vi "生成二维坐标点.vi"(1 "输入无序一维坐标点":cluster{"X":sgl, "Y":sgl}[](array[cluster])) -> (0 "输出有序二维坐标点":cluster{"X":sgl, "Y":sgl}[][](array[cluster]))   [LabVIEW 2018]
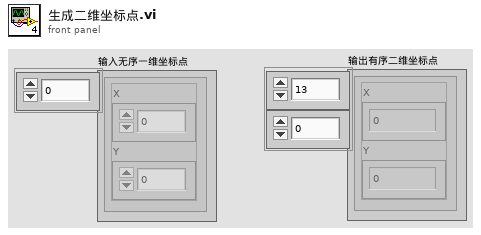
[diagram p1: front panel]
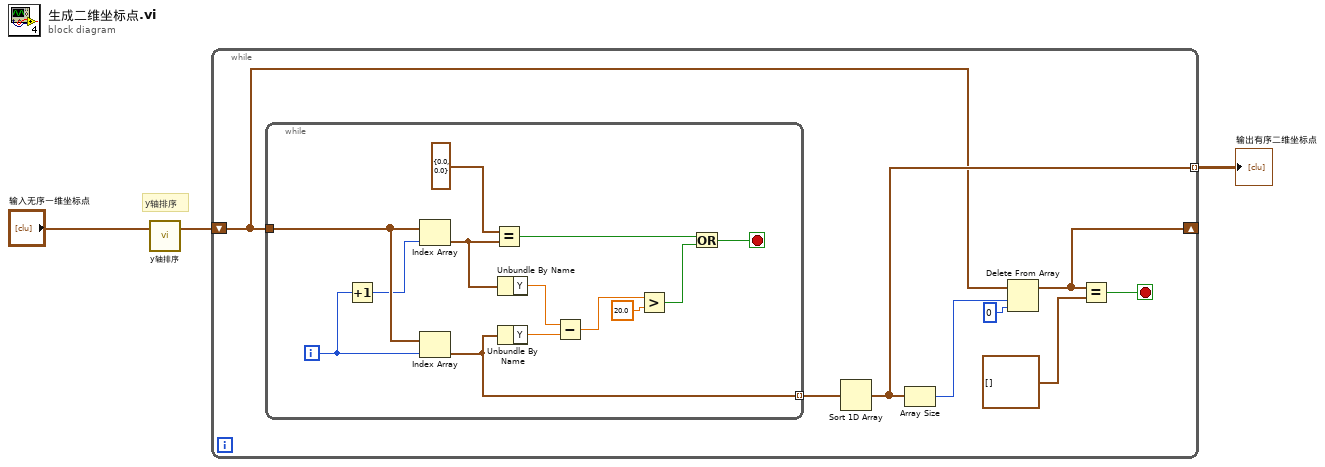
[diagram p0: block diagram]
diagram:
  # "y轴排序"
  n1 = call "y轴排序.vi"("均值角点"="输入无序一维坐标点") -> ("数组 2"=w2:cluster{"X":sgl, "Y":sgl}[])  [unwired: 2 in]
  n2 = while {
    shift-right: [w5] -> _
    shift-left: w2 -> [w4]
    tunnel: [w8] -> w3 mode=indexing
    stop <- w6 stop-if-true
    n3 = while {
      tunnel: w4 -> [w23]
      tunnel: [w19] -> w11 mode=indexing
      i -> [w24]
      stop <- w15 stop-if-true
      n4 = Increment(x=w24) -> (x+1=w22:i32)
      n5 = Index Array(array=w23, index=w22) -> (element=w14:cluster{"X":sgl, "Y":sgl})
      n6 = Index Array(array=w23, index=w24) -> (element=w19:cluster{"X":sgl, "Y":sgl})
      n7 = Equal?(x=cluster{"X":sgl, "Y":sgl} {"X"=0.0, "Y"=0.0}, y=w14) -> (x = y?=w12:bool)
      n8 = Unbundle By Name(w14) -> ("Y"=w17:sgl)
      n9 = Unbundle By Name(w19) -> ("Y"=w21:sgl)
      n10 = Subtract(x=w17, y=w21) -> (x-y=w18:sgl)
      n11 = Greater?(x=w18, y=sgl 20.0) -> (0:w16:bool)
      n12 = Or(x=w12, y=w16) -> (x .or. y?=w15:bool)
    }
    n13 = Sort 1D Array(array=w11) -> (sorted array=w8:cluster{"X":sgl, "Y":sgl}[])
    n14 = Array Size(array=w8) -> (size(s)=w10:i32)
    n15 = Delete From Array(array=w4, length=w10, index=0 ("索引")) -> (array with subset deleted=w5:cluster{"X":sgl, "Y":sgl}[])  [unwired: 1 out]
    n16 = Equal?(x=w5, y=cluster{"X":sgl, "Y":sgl}[] []) -> (x = y?=w6:bool)
  }
  "输出有序二维坐标点" <- w3
